vi "RemoveActorEnqueue.vi"(8 "error in (no error)":errorcluster, 9 "Actor's Enqueuer":refnum<class "Message Enqueuer.lvclass">, 10 "name":string, 11 "ActorMap in":refnum<class "ActorMap.lvclass">) -> (0 "error out":errorcluster, 3 "ActorMap out":refnum<class "ActorMap.lvclass">)   [LabVIEW 2020, in "ActorMap.lvclass"]
uses:
  ActorMap.lvclass
  <vilib>/ActorFramework/Message Enqueuer/Message Enqueuer.lvclass
  ActorMap.lvclass/ActorMap.ctl
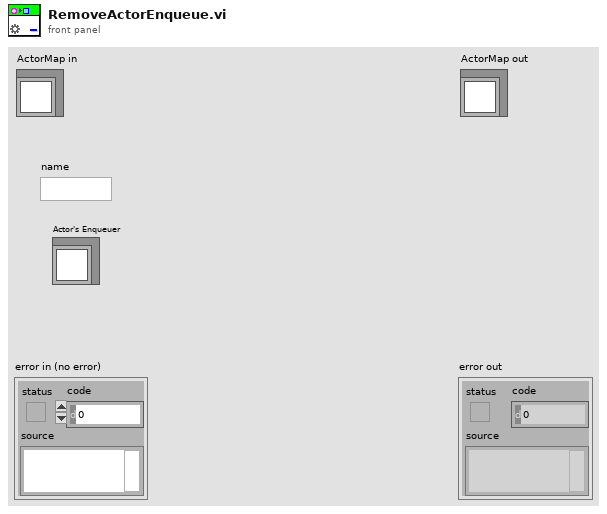
[diagram p1: front panel]
types:
  T1 = map{string, refnum<class "Message Enqueuer.lvclass">}
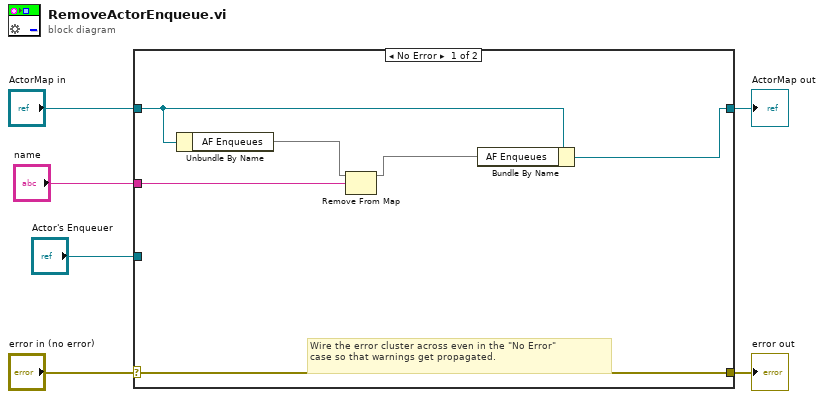
[diagram p0: block diagram]
diagram:
  n1 = case shown="No Error" "error in (no error)" {
    selector: "error in (no error)" -> [w12 w14]
    tunnel: [w12 w14] -> w5
    tunnel: [w7 w13] -> w3
    tunnel: "ActorMap in" -> [w8 w13]
    tunnel: "name" -> [w10 _]
    tunnel: "Actor's Enqueuer" -> [_ _]
    frame No Error {
      # "Wire the error cluster across even in the \"No Error\"\ncase so that warnings get propagated."
      n2 = Unbundle By Name(w8) -> ("AF Enqueues"=w11:T1)
      n3 = Remove From Map(10:w10, 11:w11) -> (3:w9:T1)  [unwired: 2 out]
      n4 = Bundle By Name(cluster=w8, "AF Enqueues"=w9) -> (w7:refnum<class "ActorMap.lvclass">)
    }
    frame Error {
    }
  }
  "error out" <- w5
  "ActorMap out" <- w3
